vi "Get_Files_in_Directory.vi"(0 "File_Names_In":string[](array[string]), 5 "File_Path":path, 11 "Error_In":errorcluster) -> (4 "File_Names_Out":string[](array[string]), 15 "Error_Out":errorcluster)   [LabVIEW 2023]
doc: "Populate instances into the tree"
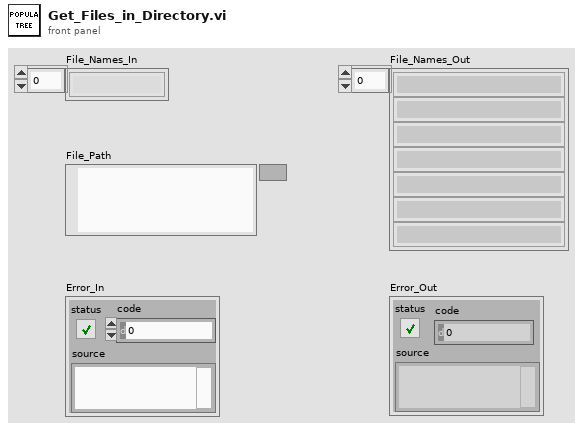
[diagram p1: front panel]
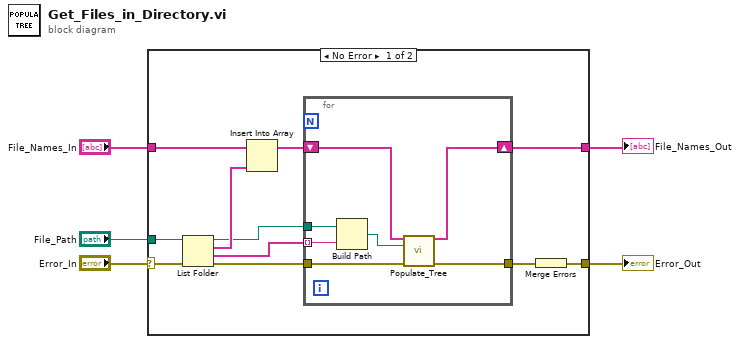
[diagram p0: block diagram]
diagram:
  n1 = case shown="No Error" "Error_In" {
    selector: "Error_In" -> [w12 w25]
    tunnel: "File_Names_In" -> [w16 w24]
    tunnel: [w13 w25] -> w4
    tunnel: "File_Path" -> [w8 _]
    tunnel: [w6 w24] -> w1
    frame No Error {
      n2 = List Folder(path=w8, error in=w12) -> (path out=w7:path, filenames=w11:string[], folder names=w9:string[], error out=w14:errorcluster)  [unwired: 2 in]
      n3 = Insert Into Array(array=w16, new element=w11) -> (w10:string[])  [unwired: 1 in]
      n4 = for {
        tunnel: w9 -> [w20] mode=indexing
        tunnel: w7 -> [w19]
        tunnel: w14 -> [w22]
        tunnel: [w23] -> w15
        shift-right: [w17] -> w6
        shift-left: w10 -> [w21]
        n5 = Build Path(base path=w19, name or relative path=w20) -> (appended path=w18:path)
        n6 = call "Populate_Tree.vi"("File_Names_In"=w21, "File_Path"=w18, "Error_In"=w22) -> ("File_Names_Out"=w17:string[], "Error_Out"=w23:errorcluster)  [unwired: 11 in]
      }
      n7 = Merge Errors(w15) -> (w13:errorcluster)
    }
    frame Error {
    }
  }
  "Error_Out" <- w4
  "File_Names_Out" <- w1
